vi "merFISH_stop_scan.vi"(7 "queue sCMOS":refnum<queue>, 8 "error in":errorcluster, 9 "BF?":bool, 10 "queue piezo":refnum<queue>, 11 "queue ASI stage":refnum<queue>) -> (0 "error out":errorcluster)   [LabVIEW 2015]
uses:
  CONTROLS/Q_ASI_stage_element.ctl
  CONTROLS/Q_MCL_piezo_element.ctl
  CONTROLS/Q_camera_element.ctl
  GLOBAL/Global_MAIN.vi
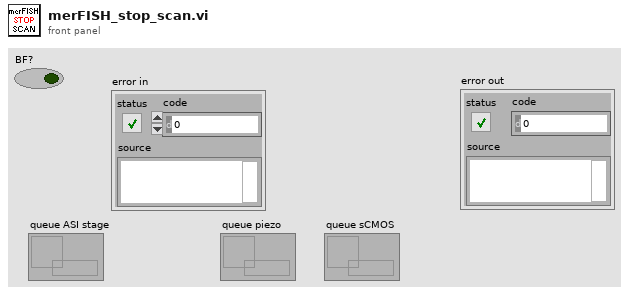
[diagram p1: front panel]
types:
  T1 = typedef "Q_camera_element.ctl" = cluster{"variant":variant, "Instruction":enum16{"CAMERA_idle", "CAMERA_initialize", "CAMERA_error", "CAMERA_security_stop", "CAMERA_not_acquiring", "CAMERA_acquiring", "CAMERA_start_acquiring", "CAMERA_stop_acquiring", "CAMERA_change_exposure", "CAMERA_define_ROI", "CAMERA_cooler", "CAMERA_acquire_movie", "CAMERA_init_scan", "CAMERA_check_new_scan_image", "CAMERA_close_scan", "CAMERA_init_merFISH", "CAMERA_start_acquiring_merFISH", "CAMERA_close_scan_merFISH", "CAMERA_close_merFISH", "CAMERA_STOP"}}
  T2 = typedef "Q_MCL_piezo_element.ctl" = cluster{"variant":variant, "Instruction":enum16{"Piezo_idle", "Piezo_initialize", "Piezo_error", "Piezo_security_stop", "Piezo_read_z", "Piezo_move_z", "Piezo_keyboard_move", "Piezo_close_autofocus_calibration_ramp", "Piezo_change_init_state", "Piezo_init_autofocus", "Piezo_init_autofocus_merFISH_TL", "Piezo_autofocus", "Piezo_autofocus_merFISH_TL", "Piezo_stop_autofocus", "Piezo_stop_autofocus_merFISH_TL", "Piezo_autofocus_lost", "Piezo_resume_autofocus_merFISH_TL", "Piezo_check_z_position_merFISH_TL", "Piezo_init_ramp", "Piezo_move_z_ramp", "Piezo_close_ramp", "Piezo_close_merFISH", "Piezo_stop"}}
  T3 = typedef "Q_ASI_stage_element.ctl" = cluster{"variant":variant, "Instruction":enum16{"ASI_idle", "ASI_initialize", "ASI_error", "ASI_security_stop", "ASI_read_XYZ", "ASI_up", "ASI_down", "ASI_left", "ASI_right", "ASI_save_XY", "ASI_move_to_XY", "ASI_brightfield", "ASI_init_scan", "ASI_init_merFISH", "ASI_move_to_XY_merFISH", "ASI_move_to_Z_merFISH", "ASI_init_autofocus_search_merFISH", "ASI_close_autofocus_search_merFISH", "ASI_adjust_piezo_autofocus_merFISH", "ASI_set_piezo_autofocus_to_reference_position_merFISH_TL", "ASI_close_merFISH", "ASI_stop"}}
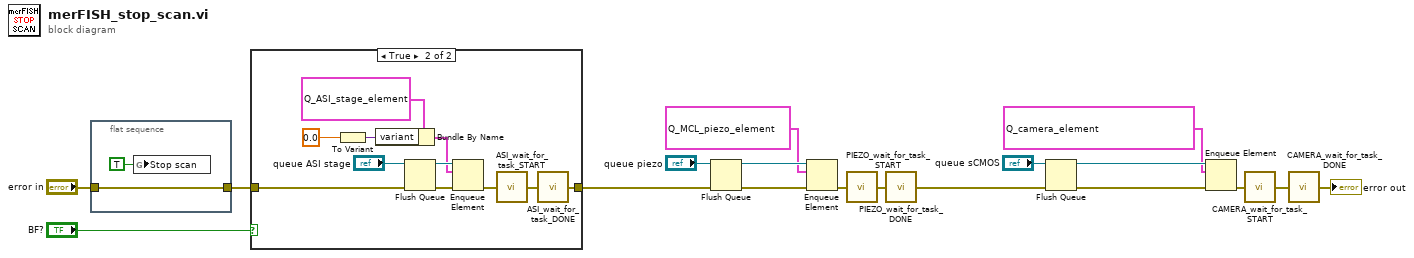
[diagram p0: block diagram]
diagram:
  n1 = flat-sequence {
    tunnel: "error in" -> [w20]
    tunnel: [w20] -> w4
    frame #0 {
      n2 = global write "Global_MAIN.vi" "Stop scan"(TRUE ("Stop scan")) -> ()
    }
  }
  n3 = case shown="True" "BF?" {
    tunnel: w4 -> [w21 w27]
    tunnel: [w21 w29] -> w16
    frame False {
    }
    frame True {
      n4 = To Variant(anything=0.0) -> (Variant=w30:variant)
      n5 = Bundle By Name(cluster=T3 {"variant"=variant, "Instruction"=enum."ASI_brightfield"} ("element"), "variant"=w30) -> (w22:T3)
      n6 = Flush Queue(queue="queue ASI stage", error in (no error)=w27) -> (queue out=w24:refnum<queue>, error out=w26:errorcluster)  [unwired: 1 out]
      n7 = Enqueue Element(queue=w24, element=w22, error in (no error)=w26) -> (error out=w31:errorcluster)  [unwired: 1 in, 2 out]
      n8 = call "ASI_wait_for_task_START.vi"("error in"=w31) -> ("error out"=w32:errorcluster)
      n9 = call "ASI_wait_for_task_DONE.vi"("error in"=w32) -> ("error out"=w29:errorcluster)
    }
  }
  n10 = Flush Queue(queue="queue piezo", error in (no error)=w16) -> (queue out=w14:refnum<queue>, error out=w17:errorcluster)  [unwired: 1 out]
  n11 = Enqueue Element(queue=w14, element=T2 {"variant"=variant, "Instruction"=enum."Piezo_close_ramp"}, error in (no error)=w17) -> (error out=w13:errorcluster)  [unwired: 1 in, 2 out]
  n12 = call "PIEZO_wait_for_task_START.vi"("error in"=w13) -> ("error out"=w12:errorcluster)
  n13 = call "PIEZO_wait_for_task_DONE.vi"("error in"=w12) -> ("error out"=w10:errorcluster)
  n14 = Flush Queue(queue="queue sCMOS", error in (no error)=w10) -> (queue out=w8:refnum<queue>, error out=w11:errorcluster)  [unwired: 1 out]
  n15 = Enqueue Element(queue=w8, element=T1 {"variant"=variant, "Instruction"=enum."CAMERA_close_scan_merFISH"}, error in (no error)=w11) -> (error out=w7:errorcluster)  [unwired: 1 in, 2 out]
  n16 = call "CAMERA_wait_for_task_START.vi"("error in"=w7) -> ("error out"=w6:errorcluster)
  n17 = call "CAMERA_wait_for_task_DONE.vi"("error in"=w6) -> ("error out"=→"error out":errorcluster)
